vi "UI.vi"() -> ()   [LabVIEW 2020]
uses:
  <vilib>/Analysis/baseanly.llb/Mean (DBL).vi
  Globals.vi
  <vilib>/Analysis/NI_AALBase.lvlib
panel:
  in  "Thermocouple Excel\nFile Location":path
  in  "Thermocouple\nExcel Button":bool
  in  "Voltage Excel\nFile Location":path
  in  "Voltage\nExcel Button":bool
  in  "Temperature Excel\nFile Location":path
  in  "Temperature \nExcel Button":bool
  out "VoltageArray":dbl[](array[numeric])
  in  "Tab Control":enum32{"Controls & Display", "Alarms"}(tab)
  out "Fahrenheit\nThermometer":dbl(slide) scale=0.0..400.0 scale format="%-#5_6g"
  out "Kelvin\nThermometer":dbl(slide)=273.0 scale=273.0..500.0 scale format="%-#5_6g"
  out "Celcius \nThermometer":dbl(slide) caption="Celcius Thermometer" scale=0.0..200.0 scale format="%-#5_6g"
  out "Temperature\nGraph 2":dbl[](graph)
  out "Temperature\nModule":dbl
  out "Voltage\nGraph":dynamicdata(graph)
  out "String":string
  out "Voltage":dbl(knob) scale=0.0..10.0
  out "F Thermocouple\nThermometer":dbl(slide) scale=0.0..400.0 scale format="%-#5_6g"
  out "K Thermocouple\nThermometer":dbl(slide) scale=273.0..500.0 scale format="%-#5_6g"
  out "C Thermocouple\nThermometer":dbl(slide) caption="Celcius Thermometer" scale=0.0..200.0 scale format="%-#5_6g"
  out "Temperature\nGraph":dbl[](graph)
  out "Thermocouple\nModule":dbl
  out "Thermocouple Alarm Led":bool
  out "Voltage Alarm Led":bool
  out "Temperature Alarm Led":bool
  in  "Thermocouple Alarm Button":bool
  in  "Voltage Alarm Button":bool
  in  "Temperature Alarm Button":bool
  in  "Thermocouple Alarm Level":dbl(slide) scale=0.0..200.0
  in  "Voltage Alarm Level":dbl(slide) scale=0.0..10.0
  in  "Temperature\nAlarm Level":dbl(slide) scale=0.0..200.0
  out "Thermocouple\nControl LED":bool
  in  "Thermocouple\nControl Switch":bool
  out "Voltage \nControl LED":bool
  in  "Voltage \nControl Switch":bool
  out "Temperature\nControl LED":bool
  in  "Temperature \nControl Switch":bool
  # "Extract to Excel"
  # "Excel location"
  # "Thermocouple\n Control"
  # "Excel location"
  # "Voltage\n Control"
  # "Excel location"
  # "Temperature\n Control"
  # "NI-9217 Temperature Values"
  # "Last:"
  # "C°"
  # "K°"
  # "F°"
  # "NI-XXXX Temperature Values"
  # "V"
  # "NI-9252 Temperature Values"
  # "Last:"
  # "C°"
  # "K°"
  # "F°"
  # "Thermocouple\nAlarm"
  # "Voltage\nAlarm"
  # "Temperature\n Alarm"
  # "ON"
  # "OFF"
  # "Thermocouple\n Control"
  # "ON"
  # "OFF"
  # "Voltage\n Control"
  # "ON"
  # "OFF"
  # "Temperature\n Control"
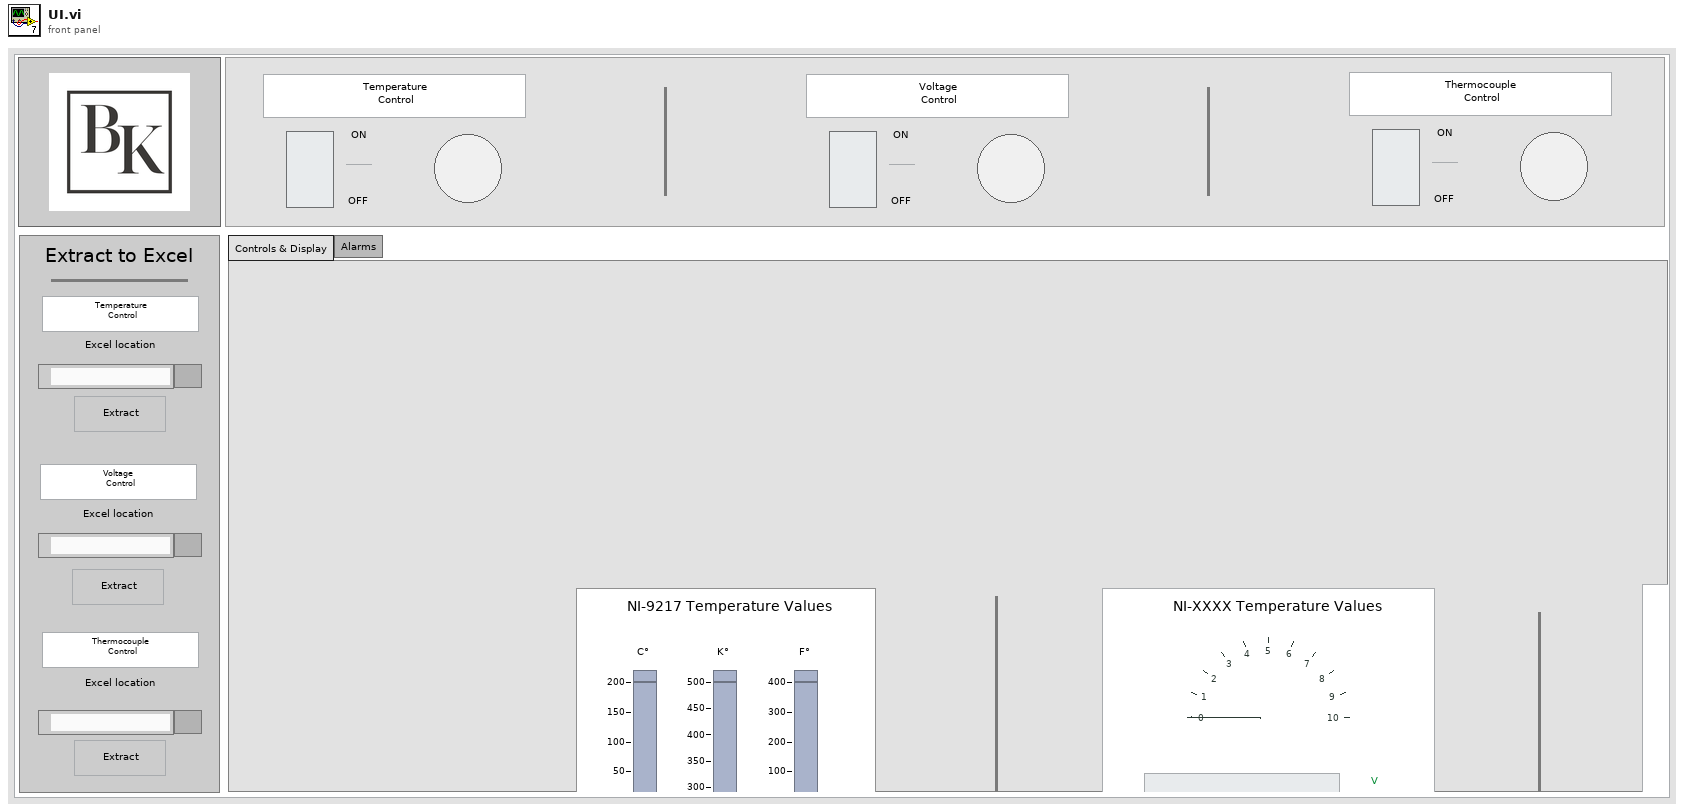
[diagram p1: front panel]
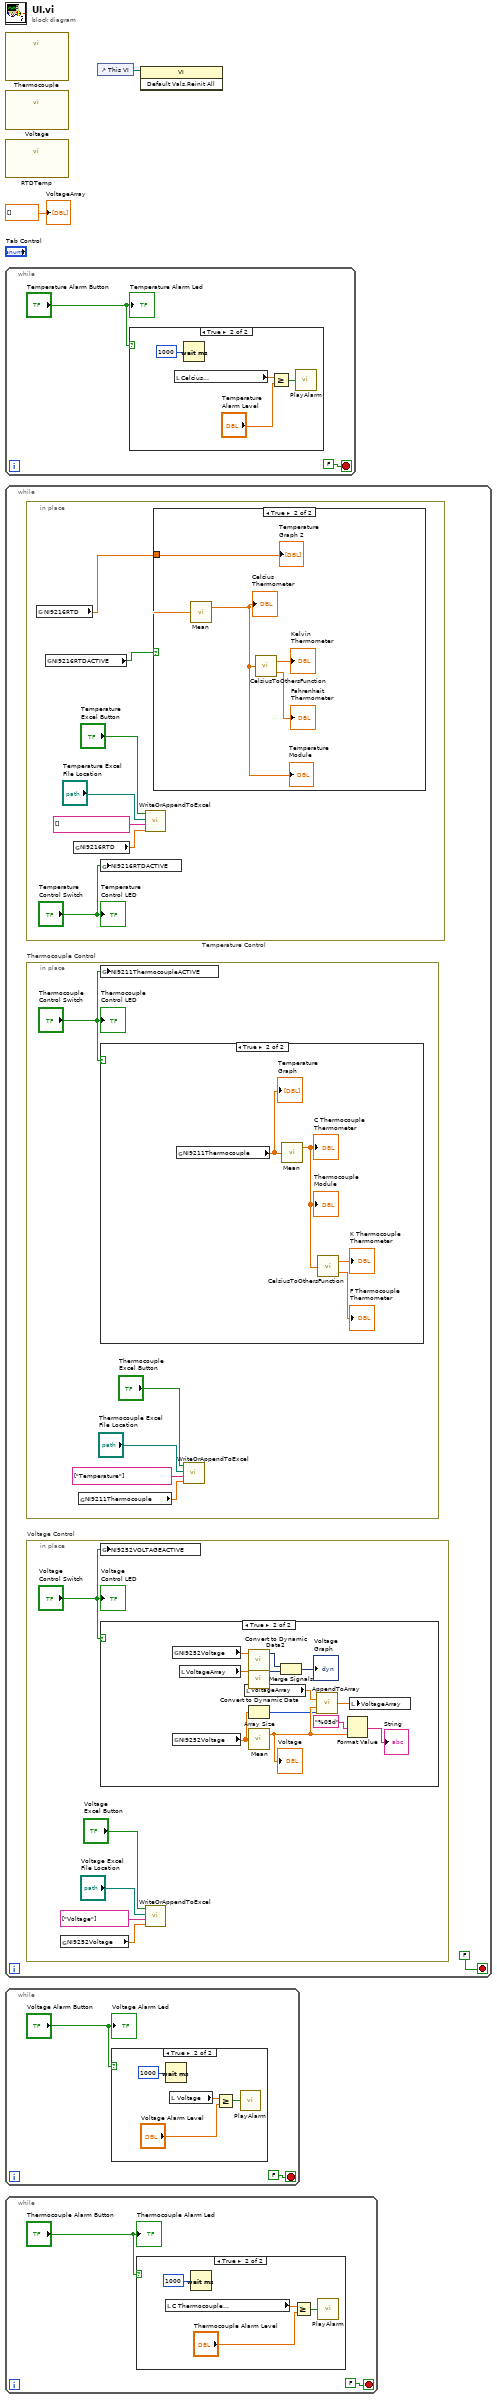
[diagram p0: block diagram]
diagram:
  n1 = call "Thermocouple.vi"() -> ()  [unwired: 12 in]
  n2 = call "Voltage.vi"() -> ()  [unwired: 12 in]
  n3 = call "RTDTemp.vi"() -> ()  [unwired: 12 in]
  n4 = while {
    stop <- FALSE stop-if-true
    n5 = case shown="True" "Temperature Alarm Button" {
      frame False {
      }
      frame True {
        n6 = local read "Celcius \nThermometer"() -> (w6:dbl)
        n7 = Wait (ms)(milliseconds to wait=u32 1000) -> ()  [unwired: 1 out]
        n8 = Greater Or Equal?(x=w6, y="Temperature\nAlarm Level") -> (x >= y?=w8:bool)
        n9 = call "PlayAlarm.vi"("Alarm Button"=w8) -> ()  [unwired: 5 in]
      }
    }
    "Temperature Alarm Led" <- "Temperature Alarm Button"
  }
  n10 = while {
    stop <- FALSE stop-if-true
    n11 = in-place "Temperature Control" {
      n12 = global read "Globals.vi" "NI9216RTD"() -> (w15:dbl[])
      n13 = global read "Globals.vi" "NI9216RTDACTIVE"() -> (w10:bool)
      n14 = global read "Globals.vi" "NI9216RTD"() -> (w11:dbl[])
      n15 = global write "Globals.vi" "NI9216RTDACTIVE"("Temperature \nControl Switch") -> ()
      n16 = call "WriteOrAppendToExcel.vi"("Data"=w11, "Column Headers"=string[] [], "Excel File Location"="Temperature Excel\nFile Location", "Excel Button"="Temperature \nExcel Button") -> ()  [unwired: 8 in]
      n17 = case shown="True" w10 {
        tunnel: w15 -> [_ w18]
        frame False {
        }
        frame True {
          n18 = call-poly <vilib>:"Mean.vi"("X"=w18) -> ("mean"=w17:dbl)  [unwired: 1 out]
          "Celcius \nThermometer" <- w17
          "Temperature\nModule" <- w17
          n19 = call "CelsiusToOthersFunction.vi"("Celsius"=w17) -> ("k"=→"Kelvin\nThermometer":dbl, "f"=→"Fahrenheit\nThermometer":dbl)
          "Temperature\nGraph 2" <- w18
        }
      }
      "Temperature\nControl LED" <- "Temperature \nControl Switch"
    }
    n20 = in-place "Thermocouple Control" {
      n21 = global read "Globals.vi" "NI9211Thermocouple"() -> (w22:dbl[])
      n22 = global write "Globals.vi" "NI9211ThermocoupleACTIVE"("Thermocouple\nControl Switch") -> ()
      n23 = case shown="True" "Thermocouple\nControl Switch" {
        frame False {
        }
        frame True {
          n24 = global read "Globals.vi" "NI9211Thermocouple"() -> (w26:dbl[])
          "Temperature\nGraph" <- w26
          n25 = call-poly <vilib>:"Mean.vi"("X"=w26) -> ("mean"=w27:dbl)  [unwired: 1 out]
          "C Thermocouple\nThermometer" <- w27
          "Thermocouple\nModule" <- w27
          n26 = call "CelsiusToOthersFunction.vi"("Celsius"=w27) -> ("k"=→"K Thermocouple\nThermometer":dbl, "f"=→"F Thermocouple\nThermometer":dbl)
        }
      }
      n27 = call "WriteOrAppendToExcel.vi"("Data"=w22, "Column Headers"=string[] ["Temperature"], "Excel File Location"="Thermocouple Excel\nFile Location", "Excel Button"="Thermocouple\nExcel Button") -> ()  [unwired: 8 in]
      "Thermocouple\nControl LED" <- "Thermocouple\nControl Switch"
    }
    n28 = in-place "Voltage Control" {
      n29 = global read "Globals.vi" "NI9252Voltage"() -> (w31:dbl[])
      n30 = global write "Globals.vi" "NI9252VOLTAGEACTIVE"("Voltage \nControl Switch") -> ()
      n31 = case shown="True" "Voltage \nControl Switch" {
        frame False {
        }
        frame True {
          n32 = global read "Globals.vi" "NI9252Voltage"() -> (w37:dbl[])
          n33 = global read "Globals.vi" "NI9252Voltage"() -> (w41:dbl[])
          n34 = local read "VoltageArray"() -> (w38:dbl[])
          n35 = local read "VoltageArray"() -> (w44:dbl[])
          n36 = call "Convert to Dynamic Data2"("Array"=w37) -> ("Dynamic Data Type"=w35:dynamicdata)  [unwired: 3 in]
          n37 = call "Convert to Dynamic Data"("Array"=w38) -> ("Dynamic Data Type"=w36:dynamicdata)  [unwired: 3 in]
          n38 = Array Size(array=w41) -> (size(s)=w40:i32)
          n39 = call-poly <vilib>:"Mean.vi"("X"=w41) -> ("mean"=w43:dbl)  [unwired: 1 out]
          "Voltage" <- w43
          n40 = Merge Signals(w35, w36) -> (→"Voltage\nGraph":dynamicdata)
          n41 = call "AppendToArray.vi"("InputArray"=w44, "Element"=w43, "MaxArraySize"=w40) -> ("OutputArray"=w42:dbl[])  [unwired: 12 in]
          n42 = Format Value(format string="%05d", value (0)=w43) -> (output string=→"String":string)  [unwired: 1 in]
          n43 = local write "VoltageArray"(w42) -> ()
        }
      }
      n44 = call "WriteOrAppendToExcel.vi"("Data"=w31, "Column Headers"=string[] ["Voltage"], "Excel File Location"="Voltage Excel\nFile Location", "Excel Button"="Voltage\nExcel Button") -> ()  [unwired: 8 in]
      "Voltage \nControl LED" <- "Voltage \nControl Switch"
    }
  }
  n45 = while {
    stop <- FALSE stop-if-true
    n46 = case shown="True" "Voltage Alarm Button" {
      frame False {
      }
      frame True {
        n47 = Wait (ms)(milliseconds to wait=u32 1000) -> ()  [unwired: 1 out]
        n48 = local read "Voltage"() -> (w51:dbl)
        n49 = Greater Or Equal?(x=w51, y="Voltage Alarm Level") -> (x >= y?=w50:bool)
        n50 = call "PlayAlarm.vi"("Alarm Button"=w50) -> ()  [unwired: 5 in]
      }
    }
    "Voltage Alarm Led" <- "Voltage Alarm Button"
  }
  n51 = while {
    stop <- FALSE stop-if-true
    n52 = case shown="True" "Thermocouple Alarm Button" {
      frame False {
      }
      frame True {
        n53 = local read "C Thermocouple\nThermometer"() -> (w57:dbl)
        n54 = Wait (ms)(milliseconds to wait=u32 1000) -> ()  [unwired: 1 out]
        n55 = Greater Or Equal?(x=w57, y="Thermocouple Alarm Level") -> (x >= y?=w56:bool)
        n56 = call "PlayAlarm.vi"("Alarm Button"=w56) -> ()  [unwired: 5 in]
      }
    }
    "Thermocouple Alarm Led" <- "Thermocouple Alarm Button"
  }
  n57 = control-ref of="This VI"() -> (w1:refnum<vi>)
  n58 = invoke class="VI" method="Default Vals.Reinit All"(reference=w1) -> ()  [unwired: 2 in, 3 out]
  "VoltageArray" <- dbl[] [] ("VoltageArray")
